vi "Wrapper.vi"(0 "Send PAS Data in":refnum<class "Send PAS Data MSG.lvclass">, 1 "Actor in":refnum<class "Actor.lvclass">, 5 "error in (no error)":errorcluster) -> (14 "Controller out":refnum<class "Controller.lvclass">, 19 "error out":errorcluster)   [LabVIEW 2014, in "Send PAS Data MSG.lvclass"]
uses:
  Send PAS Data MSG.lvclass
  Controller/Controller.lvclass
  reusable/PAS/Data/Main/PAS Data.lvclass
  Data/xData.lvclass
  <vilib>/ActorFramework/Actor/Actor.lvclass
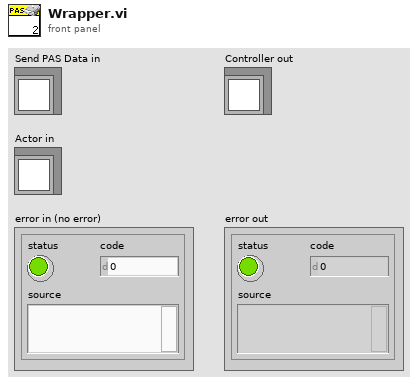
[diagram p1: front panel]
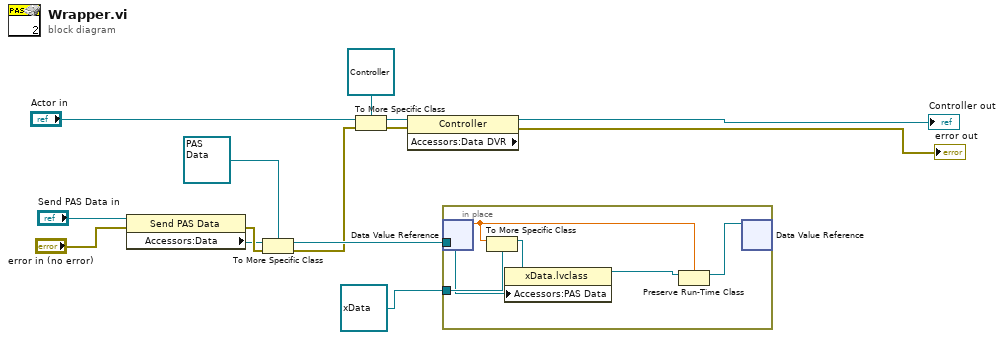
[diagram p0: block diagram]
diagram:
  n1 = property class="Send PAS Data"(reference="Send PAS Data in", error in="error in (no error)") -> (error out=w5:errorcluster, "Accessors:Data"=w3:refnum<class "Data.lvclass">)  [unwired: 1 out]
  n2 = To More Specific Class(target class=refnum<class "PAS Data.lvclass"> refnum ("PAS Data"), reference=w3, error in=w5) -> (specific class reference=w14:refnum<class "PAS Data.lvclass">, error out=w4:errorcluster)
  n3 = To More Specific Class(target class=refnum<class "Controller.lvclass"> refnum ("Controller.lvlib:Controller"), reference="Actor in", error in=w4) -> (specific class reference=w2:refnum<class "Controller.lvclass">, error out=w6:errorcluster)
  n4 = property class="Controller" props=["Accessors:Data DVR"](reference=w2, error in=w6) -> (reference out=→"Controller out":refnum<class "Controller.lvclass">, error out=→"error out":errorcluster)  [unwired: 1 out]
  n5 = in-place {
    in-place-border: refnum<class "xData.lvclass"> refnum ("xData.lvclass") -> [w20]
    in-place-border: w14 -> [w18]
    n6 = in-place-dvr #1() -> (w16:dbl)  [unwired: 1 in, 1 out]
    n7 = To More Specific Class(target class=w20, reference=w16) -> (specific class reference=w19:refnum<class "xData.lvclass">)  [unwired: 1 in, 1 out]
    n8 = property class="xData.lvclass"(reference=w19, "Accessors:PAS Data"=w18) -> (reference out=w17:refnum<class "xData.lvclass">)  [unwired: 1 in, 1 out]
    n9 = Preserve Run-Time Class(object in=w17, 2:w16) -> (object out=w15:refnum<class "Data.lvclass">)  [unwired: 1 in, 1 out]
    n10 = in-place-dvr #1(w15) -> ()  [unwired: 2 out]
  }
